vi "Event loop error handler.vi"(8 "error in (no error)":errorcluster, 9 "Next State":T1, 10 "Stop?":bool) -> (0 "error out":errorcluster, 3 "Stop event handling loop":bool)   [LabVIEW 2013]
uses:
  Typedefs/Top level VI states.ctl
  Global Variables/gl_Queues.vi
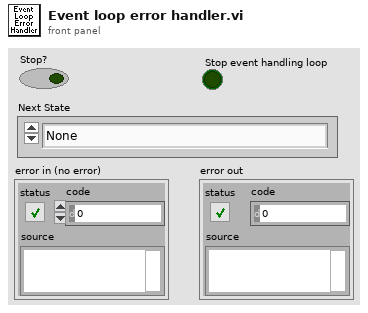
[diagram p1: front panel]
types:
  T1 = typedef "Top level VI states.ctl" = enum16{"None", "Initialise UI", "<STACK PROTOCOL STATES>", "AOL Zstack-START", "AOL Zstack-STOP", "Motor Zstack-START", "Motor Zstack-STOP", "<ACQUISITION PROTOCOL STATES> ", "Functional Acquisition-START", "Functional Acquisition-STOP", "Single Plane Acquisition-START", "Single Plane Acquisition-STOP", "Volume Acquisition-START", "Volume Acquisition-STOP", "<LIVE IMAGING PROTOCOL STATES>", "Live Imaging-START", "Live Imaging-STOP", "Live Plane Imaging-START", "Live Plane Imaging-STOP", "Live Volume Imaging-START", "Live Volume Imaging-STOP", "EXIT"}
  T2 = typedef "All Message Queues.ctl" = cluster{"UI queue":refnum<queue>, "Acq. queue":refnum<queue>, "Logging queue":refnum<queue>}
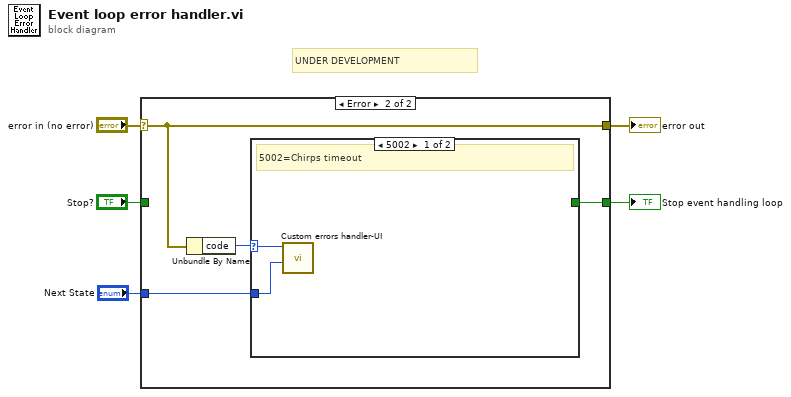
[diagram p0: block diagram]
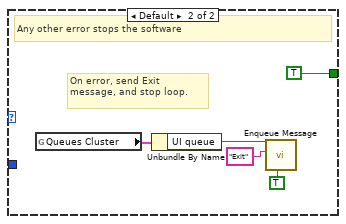
[diagram p3: hidden frame]
diagram:
  # "UNDER DEVELOPMENT"
  n1 = case shown="Error" "error in (no error)" {
    selector: "error in (no error)" -> [w7 w10]
    tunnel: [w6 w11] -> w2
    tunnel: "Stop?" -> [w6 _]
    tunnel: [w7 w10] -> w4
    tunnel: "Next State" -> [_ w8]
    frame No Error {
    }
    frame Error {
      n2 = Unbundle By Name(w10) -> ("code"=w9:i32)
      n3 = case shown="5002" w9 {
        selector: w9 -> [w13 _]
        tunnel: [_ TRUE ("Discard?")] -> w11
        tunnel: w8 -> [w12 _]
        frame 5002 {
          # "5002=Chirps timeout"
          n4 = call "Custom errors handler-UI.vi"("Next State"=w12, "code"=w13) -> ()  [unwired: 10 in]
        }
        frame Default {
          # "On error, send Exit message, and stop loop."
          # "Any other error stops the software"
          n5 = global read "gl_Queues.vi" "Queues Cluster"() -> (w15:T2)
          n6 = Unbundle By Name(w15) -> ("UI queue"=w14:refnum<queue>)
          n7 = call "Enqueue Message.vi"("Priority Message? (F)"=TRUE ("Discard?"), "Message"="Exit", "Queue"=w14) -> ()  [unwired: 7 in, 2 out]
        }
      }
    }
  }
  "error out" <- w4
  "Stop event handling loop" <- w2
